vi "cm_Set Input Ranges.vi"(0 "Display State In":T1={"Chan"=[], "First Drop?"=FALSE, "Notifier Name"="", "Refresh View"=FALSE, "Scale to Input Range"=FALSE, "Linear View"=FALSE, "Display"={"Current"=6618880, "Peak"=6618880}, "Property/Method"=enum."No Update", "Time Display Ref"=[]}, 5 "Channel Index":i32[](array[numeric]), 7 "Input Range":dbl[](array[numeric]), 9 "Container State":T3, 11 "error in (no error)":errorcluster) -> (4 "Display State Out":T1={"Chan"=[], "First Drop?"=FALSE, "Notifier Name"="", "Refresh View"=FALSE, "Scale to Input Range"=FALSE, "Linear View"=FALSE, "Display"={"Current"=6618880, "Peak"=6618880}, "Property/Method"=enum."No Update", "Time Display Ref"=[]}, 15 "error out":errorcluster)   [LabVIEW 2009, in "Channel Monitor [System].xctl"]
doc: "Set the input range for one or more channels of the Channel Monitor XControl. The default input range is 10."
uses:
  Channel Monitor [System].xctl
  <vilib>/_xctls/Container State.ctl
  subVIs/cm_Channel Monitor State.ctl
  TypeDef/cm_Property_Method.ctl
  <vilib>/_xctls/XControlSupport.lvlib
panel:
  # "Add Controls & Indicators that form the parameters of the method here. Hook them to the connector pane. Do not delete the controls & indicators that are already hooked to the connector pane.\n \nTo setup the parameters  for this method, right click on this item in the Project Tree & select \"Configure Method...\"."
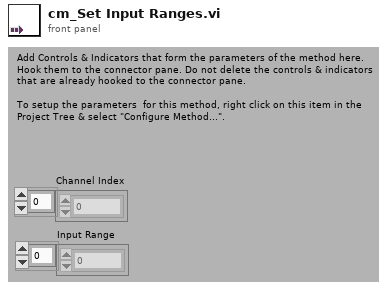
[diagram p1: front panel]
types:
  T1 = typedef "Channel Monitor [System].xctl/cm_Channel Monitor State.ctl" = cluster{"Chan":cluster{"ChanName":string, "Current":dbl, "Peak":dbl, "Input Range":dbl}[], "First Drop?":bool, "Notifier Name":string, "Refresh View":bool, "Scale to Input Range":bool, "Linear View":bool, "Display":cluster{"Current":u32, "Peak":u32}, "Property/Method":T2, "Time Display Ref":refnum<vi>[]}
  T2 = typedef "Channel Monitor [System].xctl/cm_Property_Method.ctl" = enum16{"No Update", "Color: Currrent", "Color: Peak", "Close Time Displays"}
  T3 = typedef "XControlSupport.lvlib/Container State.ctl" = cluster{"Indicator?":bool, "Run Mode?":bool, " Refnum":refnum<vi>}
  T4 = cluster{"ChanName":string, "Current":dbl, "Peak":dbl, "Input Range":dbl}[]
  T5 = cluster{"ChanName":string, "Current":dbl, "Peak":dbl, "Input Range":dbl}
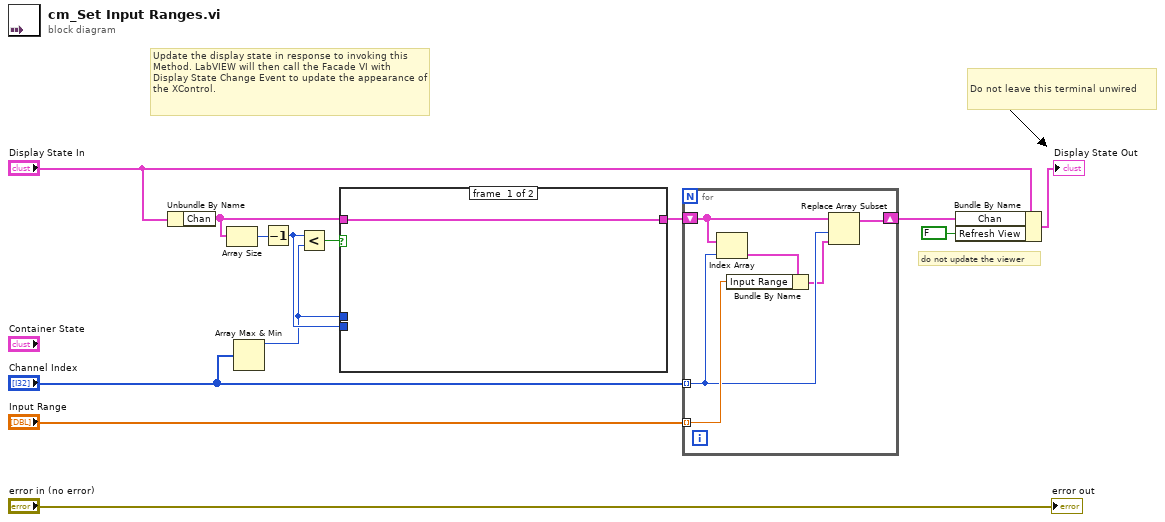
[diagram p0: block diagram]
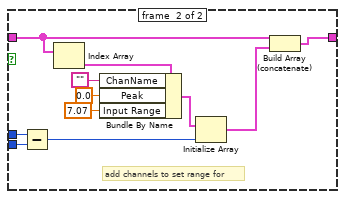
[diagram p2: hidden frame]
diagram:
  # "do not update the viewer"
  # "Do not leave this terminal unwired"
  # "Update the display state in response to invoking this Method. LabVIEW will then call the Facade VI with Display State Change Event to update the appearance of the XControl."
  n1 = Unbundle By Name("Display State In") -> ("Chan"=w8:T4)
  n2 = Array Size(array=w8) -> (size(s)=w9:i32)
  n3 = Array Max & Min(array="Channel Index") -> (max value=w5:i32)  [unwired: 3 out]
  n4 = Decrement(x=w9) -> (x-1=w6:i32)
  n5 = Less?(x=w6, y=w5) -> (x < y?=w7:bool)
  n6 = case shown="True" w7 {
    tunnel: w8 -> [w14 w17]
    tunnel: w6 -> [_ w25]
    tunnel: w5 -> [_ w24]
    tunnel: [w14 w16] -> w4
    frame #0 {
    }
    frame #1 {
      # "add channels to set range for"
      n7 = Subtract(x=w24, y=w25) -> (x-y=w18:i32)
      n8 = Index Array(array=w17) -> (element=w23:T5)  [unwired: 1 in]
      n9 = Bundle By Name(cluster=w23, "ChanName"="", "Peak"=0.0, "Input Range"=7.07) -> (w19:T5)
      n10 = Initialize Array(w19, w18) -> (w15:T4)
      n11 = Build Array (concatenate)(w17, w15) -> (w16:T4)
    }
  }
  n12 = for {
    tunnel: "Channel Index" -> [w27] mode=indexing
    tunnel: "Input Range" -> [w28] mode=indexing
    shift-right: [w31] -> w3
    shift-left: w4 -> [w30]
    n13 = Index Array(array=w30, index=w27) -> (element=w29:T5)
    n14 = Bundle By Name(cluster=w29, "Input Range"=w28) -> (w26:T5)
    n15 = Replace Array Subset(array=w30, new element=w26, index=w27) -> (w31:T4)
  }
  n16 = Bundle By Name(cluster="Display State In", "Chan"=w3, "Refresh View"=FALSE) -> (→"Display State Out":T1)
  "error out" <- "error in (no error)"
